vi "GetSampleDelay.vi"(8 "error in (no error)":errorcluster, 10 "sample rate":i32(ring)=10240 items=["102.400kS/s"=102400, "51.200kS/s"=51200, "25.600kS/s"=25600, "20.480kS/s"=20480, "12.800kS/s"=12800, "10.240kS/s"=10240, "6.400kS/s"=6400, "5.120kS/s"=5120, "4.096kS/s"=4096, "3.200kS/s"=3200, "2.560kS/s"=2560, "2.048kS/s"=2048, "1.600kS/s"=1600, "1.280kS/s"=1280, "1.024kS/s"=1024], 11 "lookup":variant) -> (0 "error out":errorcluster, 1 "delay compensation (samples)":dbl, 2 "delay compensation (OS clocks)":u32, 3 "lookup":variant)   [LabVIEW 2017, in "CmsAcquisition.lvlib"]
uses:
  <vilib>/addons/InsightCM/Devices/Shared/Cms/CmsAcquisition/CmsAcquisition.lvlib
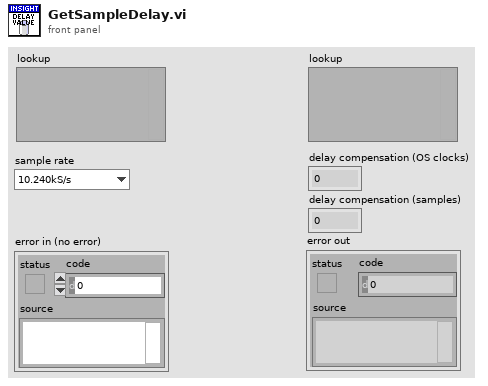
[diagram p1: front panel]
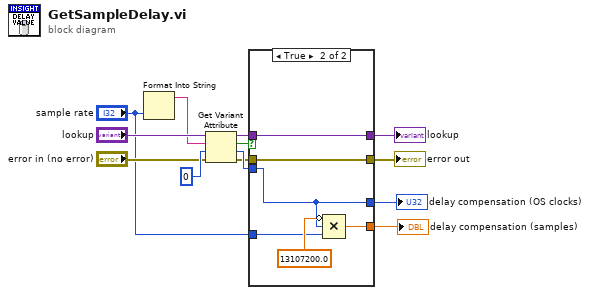
[diagram p0: block diagram]
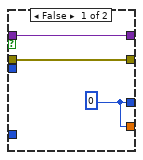
[diagram p2: hidden frame]
diagram:
  n1 = Format Into String("sample rate") -> (resulting string=w3:string)  [unwired: 3 in, 1 out]
  n2 = Get Variant Attribute(Variant="lookup", name=w3, default value (empty Variant)=u32 0, error in="error in (no error)") -> (duplicate Variant=w10:variant, found=w9:bool, value=w12:u32, error out=w5:errorcluster)
  n3 = case shown="True" w9 {
    tunnel: w10 -> [w16 w22]
    tunnel: [w16 w22] -> w11
    tunnel: w12 -> [_ w18]
    tunnel: [w14 w18] -> w13
    tunnel: w5 -> [w15 w21]
    tunnel: [w15 w21] -> w4
    tunnel: [w14 w20] -> w2
    tunnel: "sample rate" -> [_ w17]
    frame False {
      w14 = u32 0
    }
    frame True {
      n4 = Compound Arithmetic op=MULTIPLY(invert 13107200.0 ("SampClkTimebase"), w18, w17) -> (w20:dbl)
    }
  }
  "delay compensation (OS clocks)" <- w13
  "lookup" <- w11
  "error out" <- w4
  "delay compensation (samples)" <- w2
